vi "[Part 1] Process N-Channel Array.vi"() -> ()   [LabVIEW 2020]
uses:
  <vilib>/DAQmx/read.llb/DAQmx Read (Analog 1D Wfm NChan NSamp).vi
  <vilib>/DAQmx/create/channels.llb/DAQmx Create Channel (AI-Voltage-Basic).vi
  <vilib>/DAQmx/configure/timing.llb/DAQmx Timing (Sample Clock).vi
  <vilib>/DAQmx/miscellaneous.llb/DAQmx Fill In Error Info.vi
  <vilib>/measure/macond.llb/IIR Filter for N Chan.vi
  <resource>/objmgr/daqmx.rc
  <vilib>/measure/NI_MAPro.lvlib
panel:
  in  "IIR filter specifications":T1={"Topology"=enum."Butterworth", "Type"=enum."Lowpass", "Order"=1, "Lower Fc"=1.0, "Upper Fc"=200.0, "PB Ripple"=1.0, "SB Attenuation"=60.0} {"PB Ripple" format="%0.2f"; "SB Attenuation" format="%0.2f"; "Lower Fc" format="%0.2p"; "Upper Fc" format="%0.2p"}
  out "Filtered Channels":waveform(dbl)[](graph)
  out "Scaled Channels":waveform(dbl)[](graph)
  out "Actual Sample Rate (Hz)":dbl
  in  "Desired Sample Rate (Hz)":dbl=2560.0
  in  "Number of Samples":i32=256
  in  "Stop":bool
  in  "Physical Channels":tag="PCI-6221/ai0, PCI-6221/ai2:3"
  out "All Channels":waveform(dbl)[](graph)
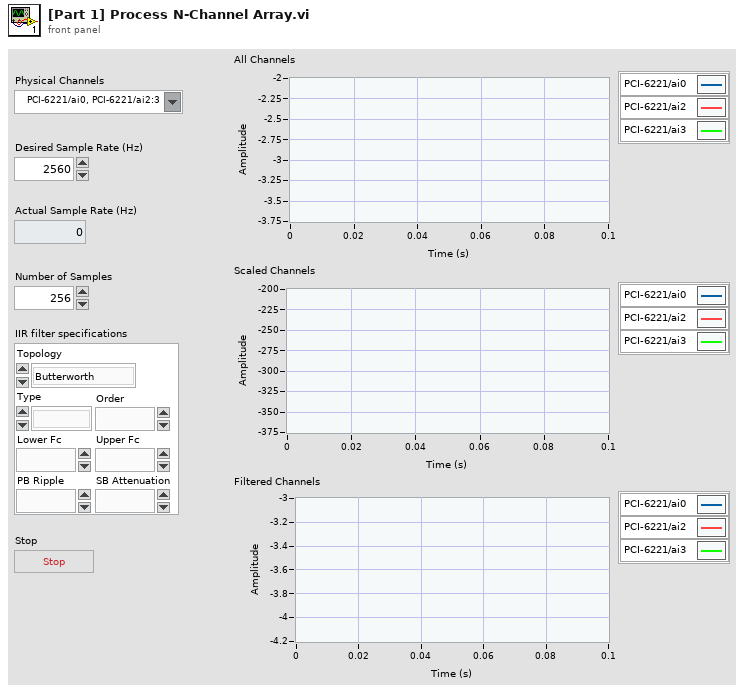
[diagram p1: front panel]
types:
  T1 = cluster{"Topology":enum16{"Off", "Butterworth", "Chebyshev", "Inverse Chebyshev", "Elliptic", "Bessel"}, "Type":enum16{"Lowpass", "Highpass", "Bandpass", "Bandstop"}, "Order":i32, "Lower Fc":dbl, "Upper Fc":dbl, "PB Ripple":dbl, "SB Attenuation":dbl}
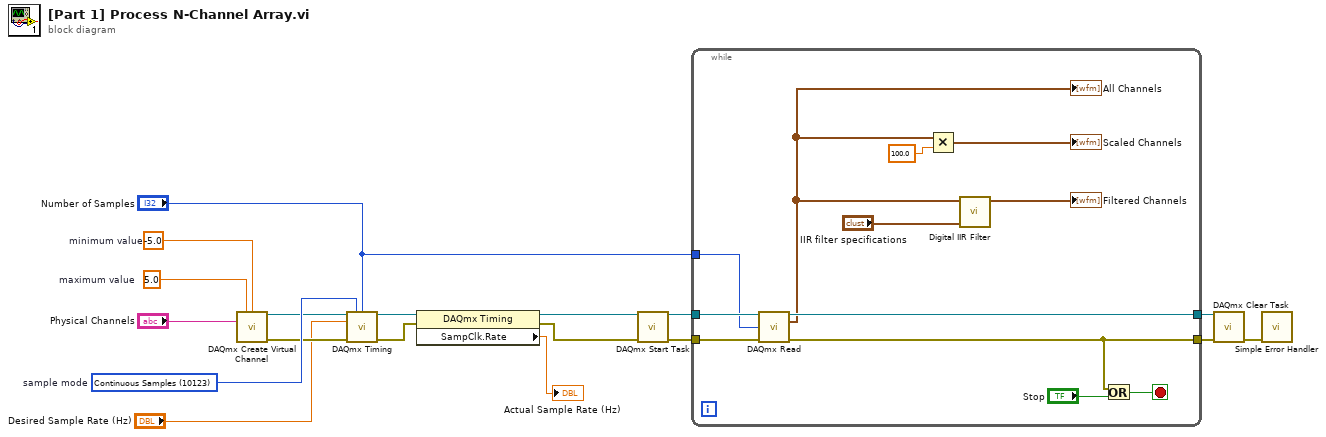
[diagram p0: block diagram]
diagram:
  w13 = 5.0  # maximum value
  w14 = -5.0  # minimum value
  w18 = 10123 items=["Finite Samples"=10178, "Continuous Samples"=10123, "Hardware Timed Single Point"=12522]  # sample mode
  n1 = call-poly <vilib>:"DAQmx Create Virtual Channel.vi"("maximum value"=w13, "minimum value"=w14, "physical channels"="Physical Channels") -> ("task out"=w17:refnum<k21>, "error out"=w16:errorcluster)  [unwired: 11 in]
  n2 = call-poly <vilib>:"DAQmx Timing.vi"("task/channels in"=w17, "sample mode"=w18, "samples per channel"="Number of Samples", "rate"="Desired Sample Rate (Hz)", "error in"=w16) -> ("task out"=w5:refnum<k21>, "error out"=w4:errorcluster)  [unwired: 9 in]
  n3 = property class="DAQmx Timing"(reference=w5, error in=w4) -> (reference out=w3:refnum<k21>, error out=w2:errorcluster, "SampClk.Rate"=→"Actual Sample Rate (Hz)":dbl)
  n4 = call <vilib>:"DAQmx Start Task.vi"("task/channels in"=w3, "error in"=w2) -> ("task out"=w9:refnum<k21>, "error out"=w8:errorcluster)  [unwired: 12 in]
  n5 = while {
    tunnel: [w30] -> w12
    tunnel: [w29] -> w11
    tunnel: w9 -> [w26]
    tunnel: w8 -> [w25]
    tunnel: "Number of Samples" -> [w24]
    stop <- w27 stop-if-true
    n6 = call-poly <vilib>:"DAQmx Read.vi"("task/channels in"=w26, "number of samples per channel"=w24, "error in"=w25) -> ("task out"=w30:refnum<k21>, "data"=w20:waveform(dbl)[], "error out"=w29:errorcluster)  [unwired: 10 in]
    "All Channels" <- w20
    n7 = Multiply(x=w20, y=100.0) -> (x*y=→"Scaled Channels":waveform(dbl)[])
    n8 = call-poly <vilib>:"Digital IIR Filter.vi"("IIR filter specifications"="IIR filter specifications", "signal(s) in"=w20) -> ("signal(s) out"=→"Filtered Channels":waveform(dbl)[])  [unwired: 7 in, 2 out]
    n9 = Or(x=w29, y="Stop") -> (x .or. y?=w27:bool)
  }
  n10 = call <vilib>:"DAQmx Clear Task.vi"("task in"=w12, "error in"=w11) -> ("error out"=w10:errorcluster)  [unwired: 13 in]
  n11 = call <vilib>:"Simple Error Handler.vi"("error in (no error)"=w10) -> ()  [unwired: 4 in, 5 out]
